vi "Resize 1d xControl.vi"(5 "Height Offset":u32, 7 "Width Offset":u32, 8 "error in (no error)":errorcluster, 10 "Control in":refnum<vi>, 11 "Pane":refnum<vi>) -> (0 "error out":errorcluster)   [LabVIEW 2011]
uses:
  Tables/XCPCCP TBL1D.xctl
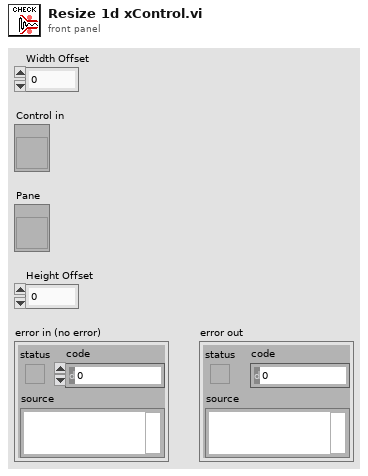
[diagram p1: front panel]
types:
  T1 = typedef "LVBoundsTypeDef.ctl" = cluster{"Width":u32, "Height":u32}
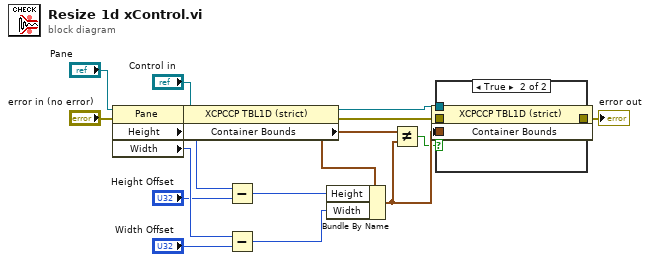
[diagram p0: block diagram]
diagram:
  n1 = property on="Property Node" class="Pane"(reference="Pane", error in="error in (no error)") -> (error out=w7:errorcluster, "Height"=w16:u32, "Width"=w15:u32)  [unwired: 1 out]
  n2 = property on="Property Node" class="XCPCCP TBL1D (strict)"(reference="Control in", error in=w7) -> (reference out=w4:refnum<vi>, error out=w8:errorcluster, "Container Bounds"=w3:T1)
  n3 = Subtract(x=w16, y="Height Offset") -> (x-y=w11:u32)
  n4 = Subtract(x=w15, y="Width Offset") -> (x-y=w14:u32)
  n5 = Bundle By Name(cluster=w3, "Height"=w11, "Width"=w14) -> (w2:T1)
  n6 = Not Equal?(x=w3, y=w2) -> (x != y?=w1:bool)
  n7 = case shown="True" w1 {
    tunnel: [w17 w21] -> w10
    tunnel: w8 -> [w17 w20]
    tunnel: w2 -> [_ w19]
    tunnel: w4 -> [_ w18]
    frame False {
    }
    frame True {
      n8 = property on="Property Node" class="XCPCCP TBL1D (strict)"(reference=w18, error in=w20, "Container Bounds"=w19) -> (error out=w21:errorcluster)  [unwired: 1 out]
    }
  }
  "error out" <- w10
